vi "draw.vi"(0 "reference":refnum<class "Graph.lvclass">, 1 "graphics":refnum<class "Graphics.lvclass">, 2 "grid":refnum<class "Grid.lvclass">, 5 "error in (no error)":errorcluster, 6 "SelectedNodes":refnum<class "AbstractNode.lvclass">[](array[class]), 7 "HideOverLays(False)":bool) -> (14 "reference out":refnum<class "Graph.lvclass">, 15 "NodesBounds":T4 {"height" format="%.2f"; "width" format="%.2f"; "y" format="%.2f"; "x" format="%.2f"}, 16 "HotSpots":T1[](array[typedef]) {"HotSpot"."y" format="%.2f"; "HotSpot"."x" format="%.2f"}, 19 "error out":errorcluster)   [LabVIEW 2014, in "Graph.lvclass"]
doc: "public void draw(Graphics2D g2, Grid g)"
uses:
  <resource>/Framework/Providers/Open_GDS/UML/Graph_class/Graph.lvclass
  <resource>/Framework/Providers/Open_GDS/UML/Graphics_class/Graphics.lvclass
  <resource>/Framework/Providers/Open_GDS/UML/Grid_class/Grid.lvclass
  <resource>/Framework/Providers/Open_GDS/UML/General/Rectangle/Rectangle Rectangle2D.ctl
  <resource>/Framework/Providers/Open_GDS/UML/AbstractNode_class/AbstractNode.lvclass
  <resource>/Framework/Providers/Open_GDS/UML/UMLEditor/UMLEditor_HotSpotData.ctl
  <resource>/Framework/Providers/Open_GDS/UML/General/Point/Point Point2D.ctl
  <resource>/Framework/Providers/Open_GDS/UML/UMLEditor/UMLEditor_HotSpotType.ctl
  <resource>/Framework/Providers/Open_GDS/UML/AbstractEdge_class/AbstractEdge.lvclass
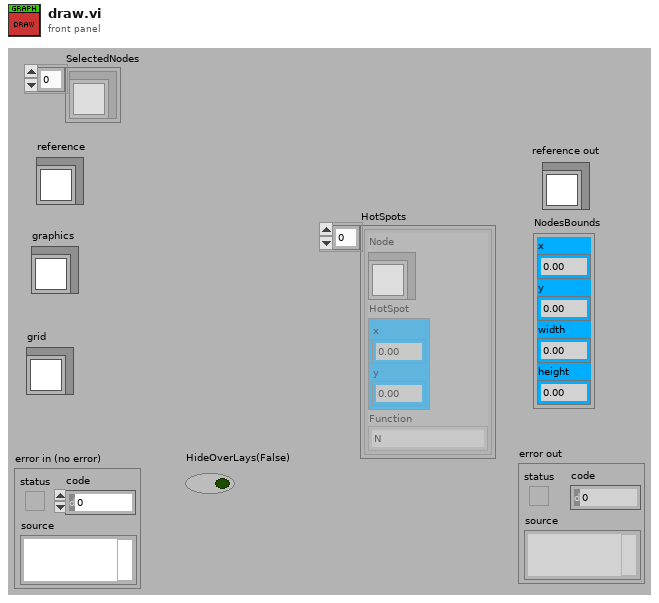
[diagram p1: front panel]
types:
  T1 = typedef "UMLEditor_HotSpotData.ctl" = cluster{"Node":refnum<class "AbstractNode.lvclass">, "HotSpot":T2, "Function":T3}
  T2 = typedef "Point Point2D.ctl" = cluster{"x":dbl, "y":dbl}
  T3 = typedef "UMLEditor_HotSpotType.ctl" = enum16{"N", "NE", "E", "SE", "S", "SW", "W", "NW", "Expand", "Collaps"}
  T4 = typedef "Rectangle Rectangle2D.ctl" = cluster{"x":dbl, "y":dbl, "width":dbl, "height":dbl}
  T5 = typedef "Graph.lvclass/ObjectAttributes.ctl" = cluster{"nodes":refnum<class "AbstractNode.lvclass">[], "edges":refnum<class "AbstractEdge.lvclass">[], "nodesToBeRemoved":refnum<class "AbstractNode.lvclass">[], "edgesToBeRemoved":refnum<class "AbstractEdge.lvclass">[], "needsLayout":bool, "LayoutNodes":refnum<class "AbstractNode.lvclass">[]}
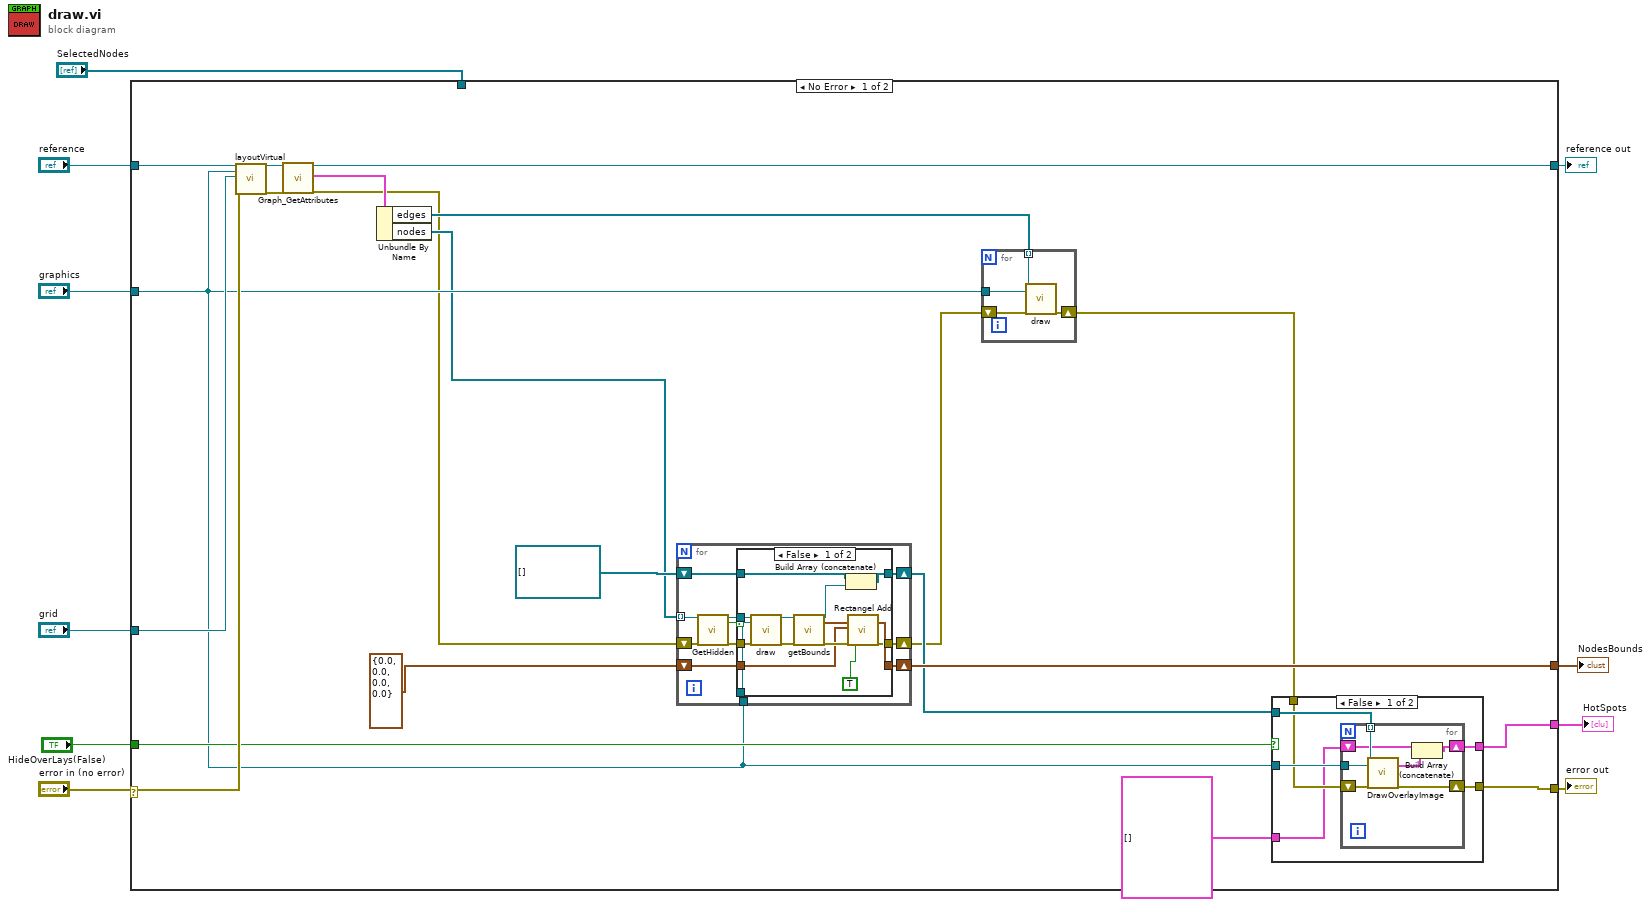
[diagram p0: block diagram]
diagram:
  n1 = case shown="No Error" "error in (no error)" {
    selector: "error in (no error)" -> [w29 w78]
    tunnel: "reference" -> [w31 w79]
    tunnel: [w14 w78] -> w9
    tunnel: [w30 w79] -> w8
    tunnel: "graphics" -> [w16 _]
    tunnel: "grid" -> [w28 _]
    tunnel: [w27 _] -> w4
    tunnel: "SelectedNodes" -> [_ _]
    tunnel: "HideOverLays(False)" -> [w21 _]
    tunnel: [w19 _] -> w1
    frame No Error {
      n2 = call <resource>:"layoutVirtual.vi"("reference"=w31, "graphics"=w16, "grid"=w28, "error in (no error)"=w29) -> ("reference out"=w24:refnum<class "Graph.lvclass">, "error out"=w23:errorcluster)  [unwired: 14 out]
      n3 = call <resource>:"Graph_GetAttributes.vi"("reference in"=w24, "error in (no error)"=w23) -> ("reference out"=w30:refnum<class "Graph.lvclass">, "Attributes"=w26:T5, "error out"=w13:errorcluster)  [unwired: 15 out]
      n4 = Unbundle By Name(w26) -> ("edges"=w25:refnum<class "AbstractEdge.lvclass">[], "nodes"=w15:refnum<class "AbstractNode.lvclass">[])
      n5 = for {
        shift-right: [w58] -> w12
        shift-left: w13 -> [w56]
        tunnel: w15 -> [w54] mode=indexing
        shift-right: [w59] -> w27
        shift-left: T4 {"x"=0.0, "y"=0.0, "width"=0.0, "height"=0.0} ("boundsAdded") -> [w60]
        tunnel: w16 -> [w57]
        shift-right: [w51] -> w18
        shift-left: refnum<class "AbstractNode.lvclass">[] [] -> [w52]
        n6 = call-dynamic "GetHidden.vi"("reference in"=w54, "error in (no error)"=w56) -> ("reference out"=w53:refnum<class "AbstractNode.lvclass">, "Hidden"=w55:bool, "error out"=w50:errorcluster)  [unwired: 15 in]
        n7 = case shown="False" w55 {
          tunnel: w60 -> [w69 w76]
          tunnel: [w68 w76] -> w59
          tunnel: [w67 w77] -> w58
          tunnel: w57 -> [w66 _]
          tunnel: w53 -> [w65 _]
          tunnel: w52 -> [w64 w75]
          tunnel: [w63 w75] -> w51
          tunnel: w50 -> [w61 w77]
          frame False {
            n8 = call-dynamic "draw.vi"("reference"=w65, "graphics"=w66, "error in (no error)"=w61) -> ("reference out"=w73:refnum<class "AbstractNode.lvclass">, "error out"=w74:errorcluster)  [unwired: 15 in]
            n9 = call-dynamic "getBounds.vi"("reference"=w73, "error in (no error)"=w74) -> ("reference out"=w62:refnum<class "AbstractNode.lvclass">, "bounds"=w72:T4, "error out"=w71:errorcluster)  [unwired: 15 in]
            n10 = Build Array (concatenate)(w64, w62) -> (w63:refnum<class "AbstractNode.lvclass">[])
            n11 = call <resource>:"Rectangel Add.vi"("bounds1"=w72, "bounds2"=w69, "error in (no error)"=w71, "useAbsoluteCordinates(False)"=TRUE) -> ("boundsAdded"=w68:T4, "error out"=w67:errorcluster)  [unwired: 1 in, 13 out]
          }
          frame True {
          }
        }
      }
      n12 = for {
        shift-right: [w46] -> w11
        shift-left: w12 -> [w49]
        tunnel: w25 -> [w47] mode=indexing
        tunnel: w16 -> [w48]
        n13 = call-dynamic "draw.vi"("reference"=w47, "graphics"=w48, "error in (no error)"=w49) -> ("error out"=w46:errorcluster)  [unwired: 15 in, 1 out]
      }
      n14 = case shown="False" w21 {
        tunnel: w16 -> [w37 _]
        tunnel: [w36 w45] -> w14
        tunnel: w18 -> [w35 _]
        tunnel: w11 -> [w34 w45]
        tunnel: T1[] [] -> [w33 _]
        tunnel: [w32 _] -> w19
        frame False {
          n15 = for {
            shift-right: [w43] -> w36
            shift-left: w34 -> [w44]
            tunnel: w35 -> [w42] mode=indexing
            tunnel: w37 -> [w41]
            shift-right: [w38] -> w32
            shift-left: w33 -> [w40]
            n16 = call-dynamic "DrawOverlayImage.vi"("reference"=w42, "graphics"=w41, "error in (no error)"=w44) -> ("HotSpots"=w39:T1[], "error out"=w43:errorcluster)  [unwired: 14 in, 1 out]
            n17 = Build Array (concatenate)(w40, w39) -> (w38:T1[])
          }
        }
        frame True {
        }
      }
    }
    frame Error {
    }
  }
  "reference out" <- w8
  "error out" <- w9
  "NodesBounds" <- w4
  "HotSpots" <- w1
